vi "create.vi"(8 "error in (no error)":errorcluster, 10 "handle":i32, 11 "client":i32) -> (0 "error out":errorcluster, 3 "RunCreateStaging out":refnum<class "RunCreateStaging.lvclass">)   [LabVIEW 2020, in "RunCreateStaging.lvclass"]
uses:
  RunCreateStaging.lvclass
  RunCreateStaging.lvclass/RunCreateStaging.ctl
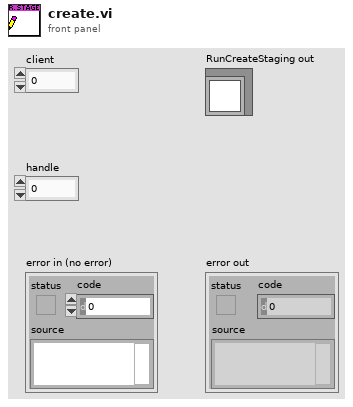
[diagram p1: front panel]
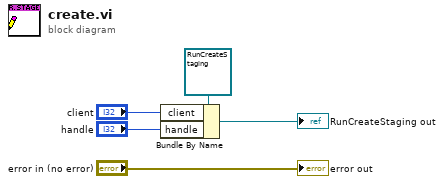
[diagram p0: block diagram]
diagram:
  n1 = Bundle By Name(cluster=refnum<class "RunCreateStaging.lvclass"> refnum ("RunCreateStaging out"), "client"="client", "handle"="handle") -> (→"RunCreateStaging out":refnum<class "RunCreateStaging.lvclass">)
  "error out" <- "error in (no error)"
